vi "user32_ArrangeIconicWindows.vi"(0 "hWnd":u32, 11 "错误输入（无错误）":errorcluster) -> (4 "dup hWnd":u32, 6 "success?":bool, 8 "IconHeight":u32, 15 "错误输出":errorcluster)   [LabVIEW 2011]
doc: "排列一个父窗口的最小化子窗口。"
uses:
  user32.dll
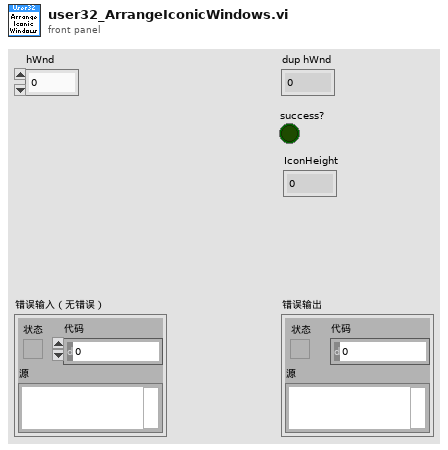
[diagram p1: front panel]
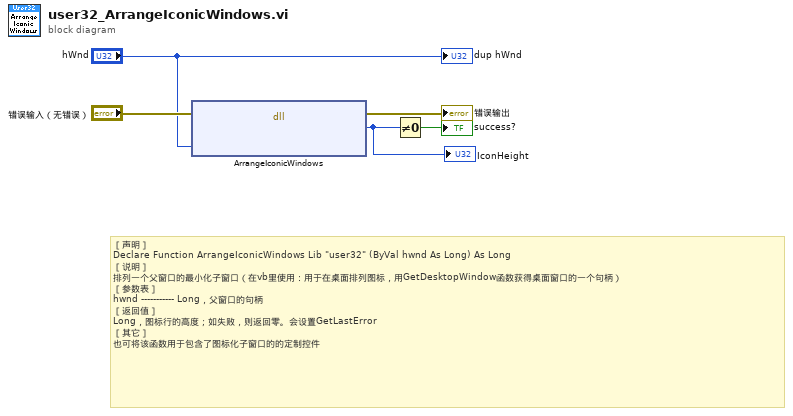
[diagram p0: block diagram]
diagram:
  # "［声明］\nDeclare Function ArrangeIconicWindows Lib \"user32\" (ByVal hwnd As Long) As Long\n［说明］\n排列一个父窗口的最小化子窗口（在vb里使用：用于在桌面排列图标，用GetDesktopWindow函数获得桌面窗口的一个句柄）\n［参数表］\nhwnd ----------- Long，父窗口的句柄\n［返回值］\nLong，图标行的高度；如失败，则返回零。会设置GetLastError\n［其它］\n也可将该函数用于包含了图标化子窗口的的定制控件"
  n1 = dll-call lib="user32.dll" fn="ArrangeIconicWindows"(error in="错误输入（无错误）", "hWnd"="hWnd") -> (error out=→"错误输出":errorcluster, "Long"=w2:u32)  [unwired: 3 in, 1 out]
  "IconHeight" <- w2
  n2 = Not Equal To 0?(x=w2) -> (x != 0?=→"success?":bool)
  "dup hWnd" <- "hWnd"
